vi "LVClass Probe.vi"(11 "LabVIEW Object":refnum<class>) -> (2 "Value String":string, 3 "Boolean":bool)   [LabVIEW 2017]
uses:
  <vilib>/Utility/Data Type/NI_Data Type.lvlib
panel:
  out "Display string":string
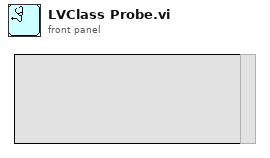
[diagram p1: front panel]
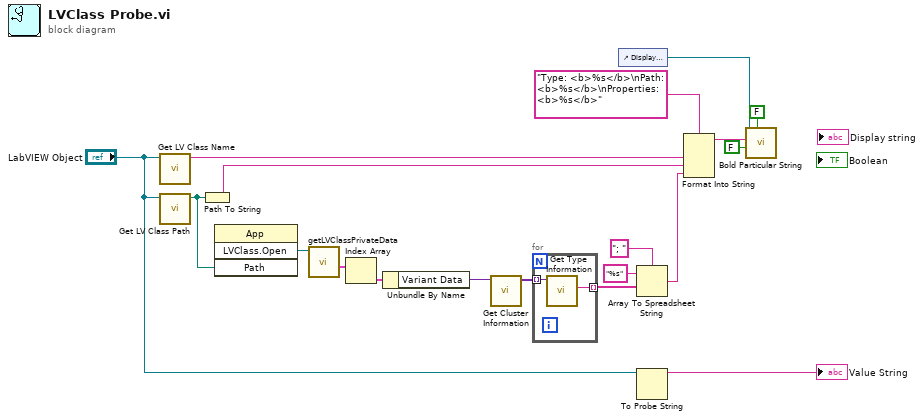
[diagram p0: block diagram]
diagram:
  n1 = call <vilib>:"Get LV Class Name.vi"("object"="LabVIEW Object") -> ("class name"=w9:string)  [unwired: 9 in, 1 out]
  n2 = call <vilib>:"Get LV Class Path.vi"("object"="LabVIEW Object") -> ("class path"=w8:path)  [unwired: 9 in, 1 out]
  n3 = Path To String(path=w8) -> (string=w13:string)
  n4 = invoke class="App" method="LVClass.Open"("Path"=w8) -> ("LVClass.Open"=w7:refnum<vi>)  [unwired: 3 in, 3 out]
  n5 = call "getLVClassPrivateData.vi"("LVClass refnum"=w7) -> ("Class Private Data Values"=w6:cluster{"Name":string, "Variant Data":variant}[])  [unwired: 7 in, 3 out]
  n6 = Index Array(array=w6) -> (element=w5:cluster{"Name":string, "Variant Data":variant})  [unwired: 1 in]
  n7 = Unbundle By Name(w5) -> ("Variant Data"=w4:variant)
  n8 = call <vilib>:"Get Cluster Information.vi"("Variant"=w4) -> ("Cluster Elements"=w3:variant[])  [unwired: 9 in, 1 out]
  n9 = for {
    tunnel: w3 -> [w21] mode=indexing
    tunnel: [w20] -> w2 mode=indexing
    n10 = call <vilib>:"Get Type Information.vi"("Variant"=w21) -> ("Name"=w20:string)  [unwired: 6 in, 4 out]
  }
  n11 = control-ref of="Display string"() -> (w16:refnum<vi>)
  n12 = Array To Spreadsheet String(delimiter (Tab)="; ", array=w2, 3:"%s" ("format string")) -> (spreadsheet string=w11:string)
  n13 = To Probe String(7:"LabVIEW Object") -> (3:→"Value String":string)  [unwired: 2 in, 1 out]
  n14 = Format Into String(format string="Type: <b>%s</b>\nPath: <b>%s</b>\nProperties: <b>%s</b>", w9, w13, w11) -> (resulting string=w17:string)  [unwired: 2 in, 1 out]
  n15 = call <vilib>:"Bold Particular String.vi"("Always Refresh? (TRUE)"=FALSE, "resize string? (TRUE)"=FALSE, "text to display"=w17, "string refnum"=w16) -> ()  [unwired: 6 in, 2 out]
